vi "Read Connected Clients ListBox Ref.vi"(11 "Function in":refnum<class "Function.lvclass">) -> (2 "Connected Clients":refnum<vi>, 3 "Function out":refnum<class "Function.lvclass">)   [LabVIEW 2016, in "Function Actor.lvlib" / "Function.lvclass"]
uses:
  <userlib>/Common Components/Function Actor/Function.lvclass
  <userlib>/Common Components/Function Actor/Function.lvclass/Function.ctl
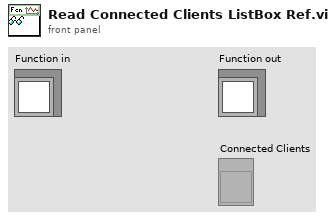
[diagram p1: front panel]
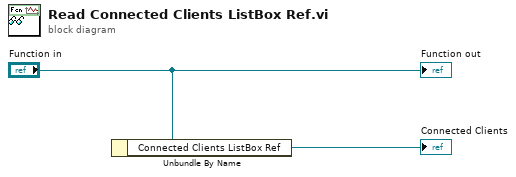
[diagram p0: block diagram]
diagram:
  n1 = Unbundle By Name("Function in") -> ("Connected Clients ListBox Ref"=→"Connected Clients":refnum<vi>)
  "Function out" <- "Function in"
